vi "GetTimeout_5782.vi"(11 "scope in":T1) -> (1 "Time left":i32, 3 "scope out":T1)   [LabVIEW 2013]
uses:
  controls/scope_params_5782.ctl
  Utilities/Ticker/Ticker.lvclass
  Communication/Driver/RemoteConnection/RemoteConnection.lvclass
  Scope/controls/ScopeMode.ctl
  Config/FPGAref_5782.ctl
  FPGA/DataMode.ctl
  controls/5782_trigger_type.ctl
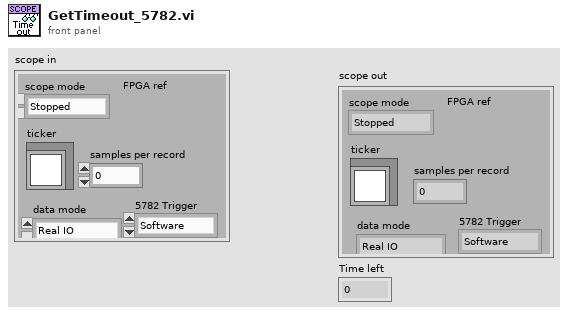
[diagram p1: front panel]
types:
  T1 = typedef "scope_params_5782.ctl" = cluster{"scope mode":T2, "ticker":refnum<class "Ticker.lvclass">, "samples per record":i32, "FPGA ref":T3, "data mode":T4, "5782 Trigger":T5, "Chart length":i32, "RemoteConnection":refnum<class "RemoteConnection.lvclass">, "last phase":dbl[]}
  T2 = typedef "ScopeMode.ctl" = enum16{"Stopped", "Single", "Running", "Continuous"}
  T3 = typedef "FPGAref_5782.ctl" = refnum<k20>
  T4 = typedef "DataMode.ctl" = enum16{"Real IO", "Simulated"}
  T5 = typedef "5782_trigger_type.ctl" = enum16{"Software", "Trigger input"}
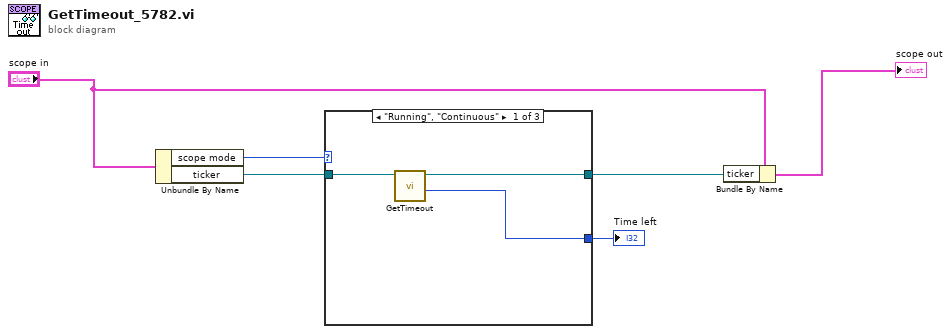
[diagram p0: block diagram]
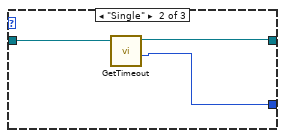
[diagram p2: hidden frame]
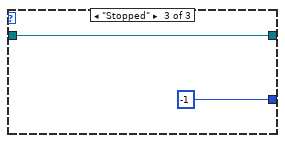
[diagram p3: hidden frame]
diagram:
  n1 = Unbundle By Name("scope in") -> ("scope mode"=w6:T2, "ticker"=w5:refnum<class "Ticker.lvclass">)
  n2 = case shown="\"Running\", \"Continuous\"" w6 {
    tunnel: w5 -> [w9 w12 w13]
    tunnel: [w8 w10 -1 ("Time left")] -> w4
    tunnel: [w7 w11 w13] -> w2
    frame "Running", "Continuous" {
      n3 = call "GetTimeout.vi"("Ticker In"=w9) -> ("Time left"=w8:i32, "Ticker Out"=w7:refnum<class "Ticker.lvclass">)  [unwired: 7 in, 2 out]
    }
    frame "Single" {
      n4 = call "GetTimeout.vi"("Ticker In"=w12) -> ("Time left"=w10:i32, "Ticker Out"=w11:refnum<class "Ticker.lvclass">)  [unwired: 7 in, 2 out]
    }
    frame "Stopped" {
    }
  }
  "Time left" <- w4
  n5 = Bundle By Name(cluster="scope in", "ticker"=w2) -> (→"scope out":T1)
